vi "KE622x -- Set Voltage Limit.vi"(0 "Resource In":refnum<visa-resource-name>, 1 "Check For SCPI Errors? (T)":bool=TRUE, 7 "Voltage Limit (V)":T1=10.0 min=0.1 max=105.0 step=0.01 format="%.2p", 11 "error in (no error)":errorcluster) -> (4 "Resource Out (dupl)":refnum<visa-resource-name>, 15 "error out":errorcluster)   [LabVIEW 2020, in "Keithley 622x.lvlib"]
doc: "Sets the voltage limit (compliance) for the current source."
uses:
  Keithley 622x.lvlib
  Typedefs/KE622x -- Voltage Limit.ctl
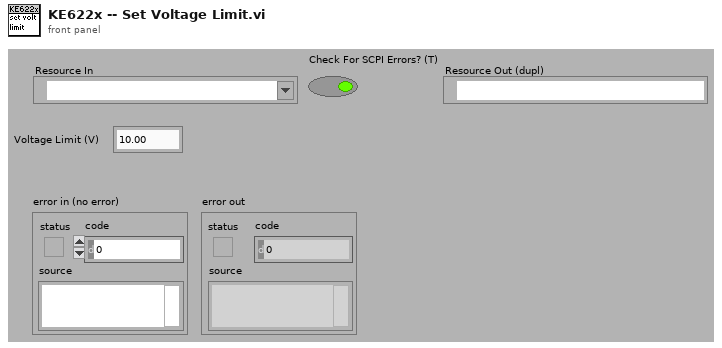
[diagram p1: front panel]
types:
  T1 = typedef "Keithley 622x.lvlib/KE622x -- Voltage Limit.ctl" = dbl
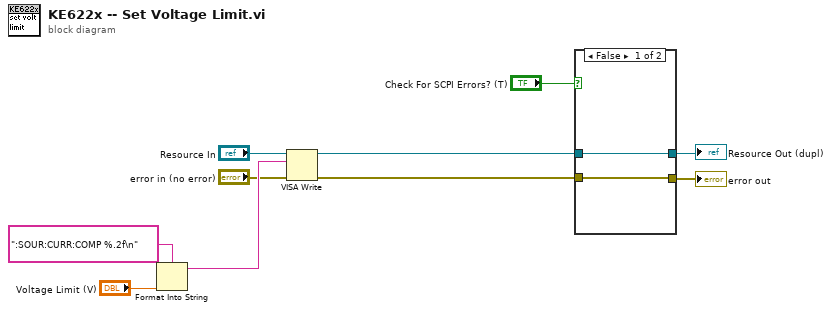
[diagram p0: block diagram]
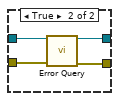
[diagram p2: hidden frame]
diagram:
  n1 = Format Into String(format string=":SOUR:CURR:COMP %.2f\n", "Voltage Limit (V)") -> (resulting string=w7:string)  [unwired: 2 in, 1 out]
  n2 = VISA Write(VISA resource name="Resource In", write buffer=w7, error in (no error)="error in (no error)") -> (VISA resource name out=w4:refnum<visa-resource-name>, error out=w3:errorcluster)  [unwired: 1 out]
  n3 = case shown="False" "Check For SCPI Errors? (T)" {
    tunnel: w4 -> [w12 w16]
    tunnel: w3 -> [w11 w15]
    tunnel: [w11 w14] -> w1
    tunnel: [w12 w13] -> w2
    frame False {
    }
    frame True {
      n4 = call "Error Query.vi"("VISA Resource In"=w16, "error in (no error)"=w15) -> ("VISA Resource Out (dupl)"=w13:refnum<visa-resource-name>, "error out"=w14:errorcluster)  [unwired: 10 in, 2 out]
    }
  }
  "Resource Out (dupl)" <- w2
  "error out" <- w1
